vi "Auto Save Trigger Data.vi"(0 "Samples Recorded":u32 format="%#.0f", 1 "Data Log Indicies":i32[](array[numeric]), 2 "Log Path Ref":refnum<file>, 3 "Config":T1={"DAQ Settings"={"Trigger Type"=enum."Manual", "Trigger Samples"=0, "Pretrigger Samples"=0, "Trigger Interval"=0.0, "Time Units"=FALSE, "Auto Save"=FALSE, "Sample Rate"=7.0, "Select Analog"=FALSE, "Trigger Value"=0.0, "Trigger Stop Method"=enum."Use Samples Value to Stop Trigger", "Rate Sec/Min"=FALSE, "Save Mode"=enum."Single File", "File Size Limit"=0.0, "Log File Type"=enum."Basic", "Trigger Data Index"=0, "Log Rate"=7.0, "Rate Sec/Min (Log)"=FALSE, "Sample Rate (S/s)"=0.0, "Log Rate (S/s)"=0.0}, "Channels"=[], "Header"={"CA Number"="", "Test Name"="", "Serial Number"="", "Technician"=""}, "Graph Settings"={"Graph Labels"=[], [], [], [], [], [], [], [], [], [], [], [], [], "Graph Toggles"=[], "Axis Toggles"=[], "Graph Range"=enum."1"}, "Test Limits"=[], "All Type Info"=[], "Save Mode"=enum."Single File", "Data Base Path"=path ""} {"DAQ Settings"."Trigger Interval" min=0.0; "DAQ Settings"."Pretrigger Samples" min=0; "DAQ Settings"."Trigger Samples" min=0}, 4 "Data":sgl[][](array[numeric]), 5 "Start Time":timestamp, 6 "Add Data Point":bool, 7 "Samples Acquired":u32, 11 "Pretrigger Size":i32) -> (14 "Samples Recorded OUT":u32, 18 "Stop DAQ":bool, 19 "Samples Acquired OUT":u32)   [LabVIEW 2023]
uses:
  Type Defs and Controls/Sensor Config.ctl
  Type Defs and Controls/DAQ Settings.ctl
  Type Defs and Controls/Trigger Stop Method.ctl
  Type Defs and Controls/Log File Type.ctl
  Type Defs and Controls/Channel Config.ctl
  Type Defs and Controls/Header.ctl
  Type Defs and Controls/Graph Settings Type Def.ctl
  Type Defs and Controls/Test Limits.ctl
  Type Defs and Controls/All Part Info.ctl
  Type Defs and Controls/Part Info.ctl
panel:
  # "EGU"
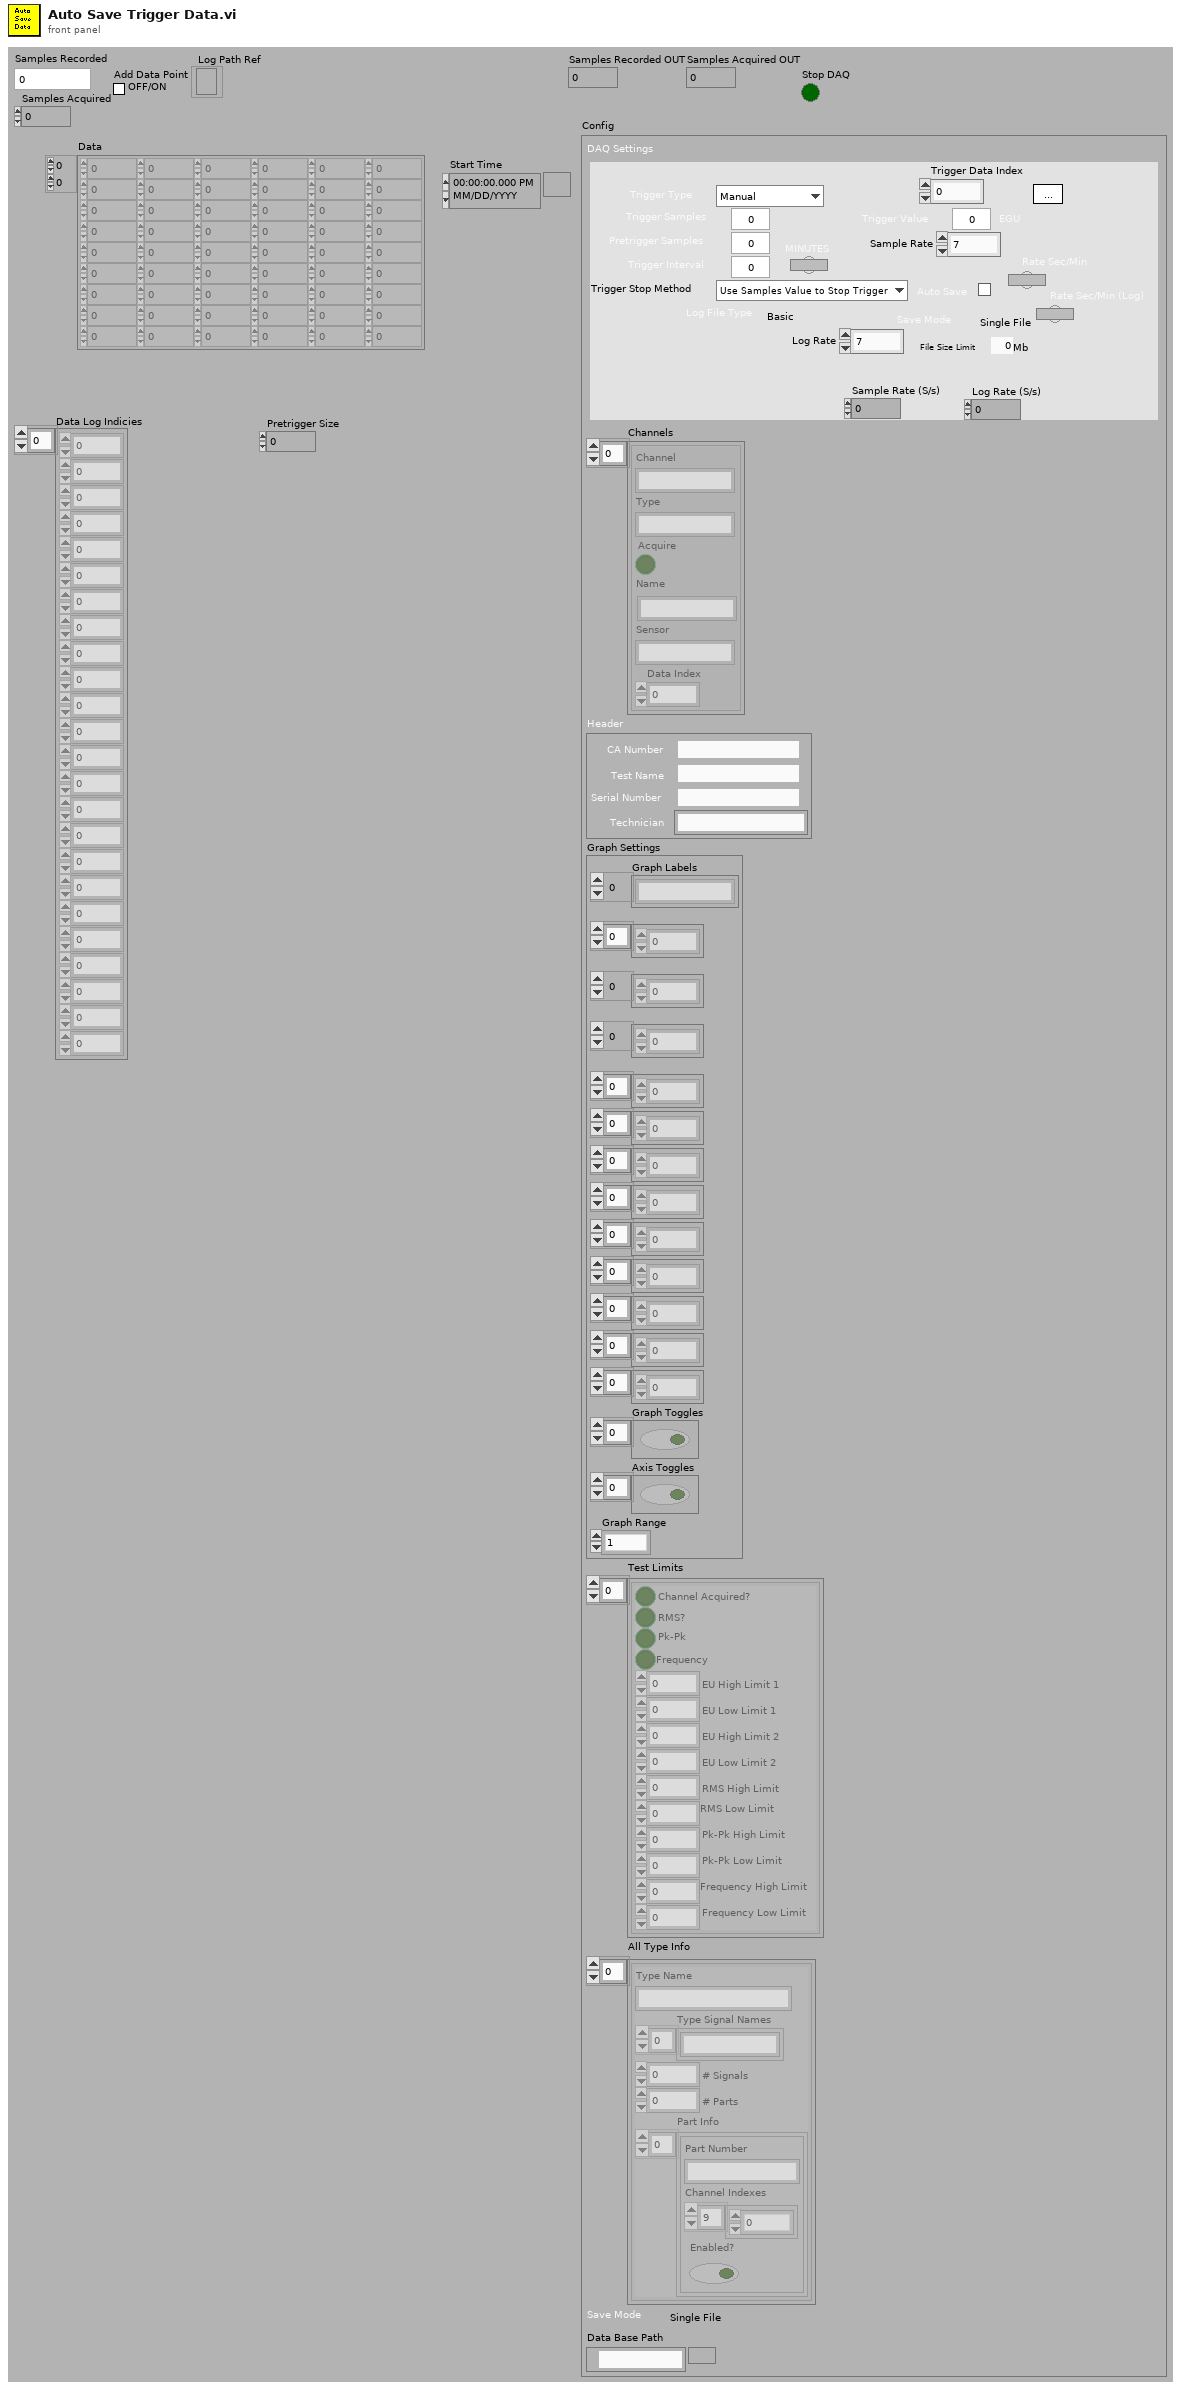
[diagram p1: front panel]
types:
  T1 = typedef "Sensor Config.ctl" = cluster{"DAQ Settings":T2, "Channels":T5[], "Header":T6, "Graph Settings":T7, "Test Limits":T8[], "All Type Info":T9, "Save Mode":enum16{"Single File", "Segmented Files", "New File at Midnight"}, "Data Base Path":path}
  T2 = typedef "DAQ Settings.ctl" = cluster{"Trigger Type":enum16{"Manual", "Timed", "Analog Rising", "Analog Falling"}, "Trigger Samples":i32, "Pretrigger Samples":i32, "Trigger Interval":dbl, "Time Units":bool, "Auto Save":bool, "Sample Rate":dbl, "Select Analog":bool, "Trigger Value":dbl, "Trigger Stop Method":T3, "Rate Sec/Min":bool, "Save Mode":enum16{"Single File", "Segmented Files", "New File at Midnight"}, "File Size Limit":dbl, "Log File Type":T4, "Trigger Data Index":u32, "Log Rate":dbl, "Rate Sec/Min (Log)":bool, "Sample Rate (S/s)":dbl, "Log Rate (S/s)":dbl}
  T3 = typedef "Trigger Stop Method.ctl" = enum16{"Use Samples Value to Stop Trigger", "Use Threshold to Stop Trigger"}
  T4 = typedef "Log File Type.ctl" = enum16{"Basic", "RTS"}
  T5 = typedef "Channel Config.ctl" = cluster{"Channel":string, "Type":string, "Acquire":bool, "Name":string, "Sensor":string, "Data Index":u32}
  T6 = typedef "Header.ctl" = cluster{"CA Number":string, "Test Name":string, "Serial Number":string, "Technician":string}
  T7 = typedef "Graph Settings Type Def.ctl" = cluster{"Graph Labels":string[], u8[], i16[], u32[], u8[], u8[], u8[], u32[], u8[], u8[], u8[], dbl[], dbl[], "Graph Toggles":bool[], "Axis Toggles":bool[], "Graph Range":enum16{"1", "2", "3", "4", "5", "10", "15", "30", "60"}}
  T8 = typedef "Test Limits.ctl" = cluster{"Channel Acquired?":bool, "RMS?":bool, "Pk-Pk":bool, "Frequency":bool, "EU High Limit 1":dbl, "EU Low Limit 1":dbl, "EU High Limit 2":dbl, "EU Low Limit 2":dbl, "RMS High Limit":dbl, "RMS Low Limit":dbl, "Pk-Pk High Limit ":dbl, "Pk-Pk Low Limit":dbl, "Frequency High Limit":dbl, "Frequency Low Limit":dbl}
  T9 = typedef "All Part Info.ctl" = cluster{"Type Name":string, "Type Signal Names":string[], "# Signals":i32, "# Parts":i32, "Part Info":T10[]}[]
  T10 = typedef "Part Info.ctl" = cluster{"Part Number":string, "Channel Indexes":u16[], "Enabled?":bool}
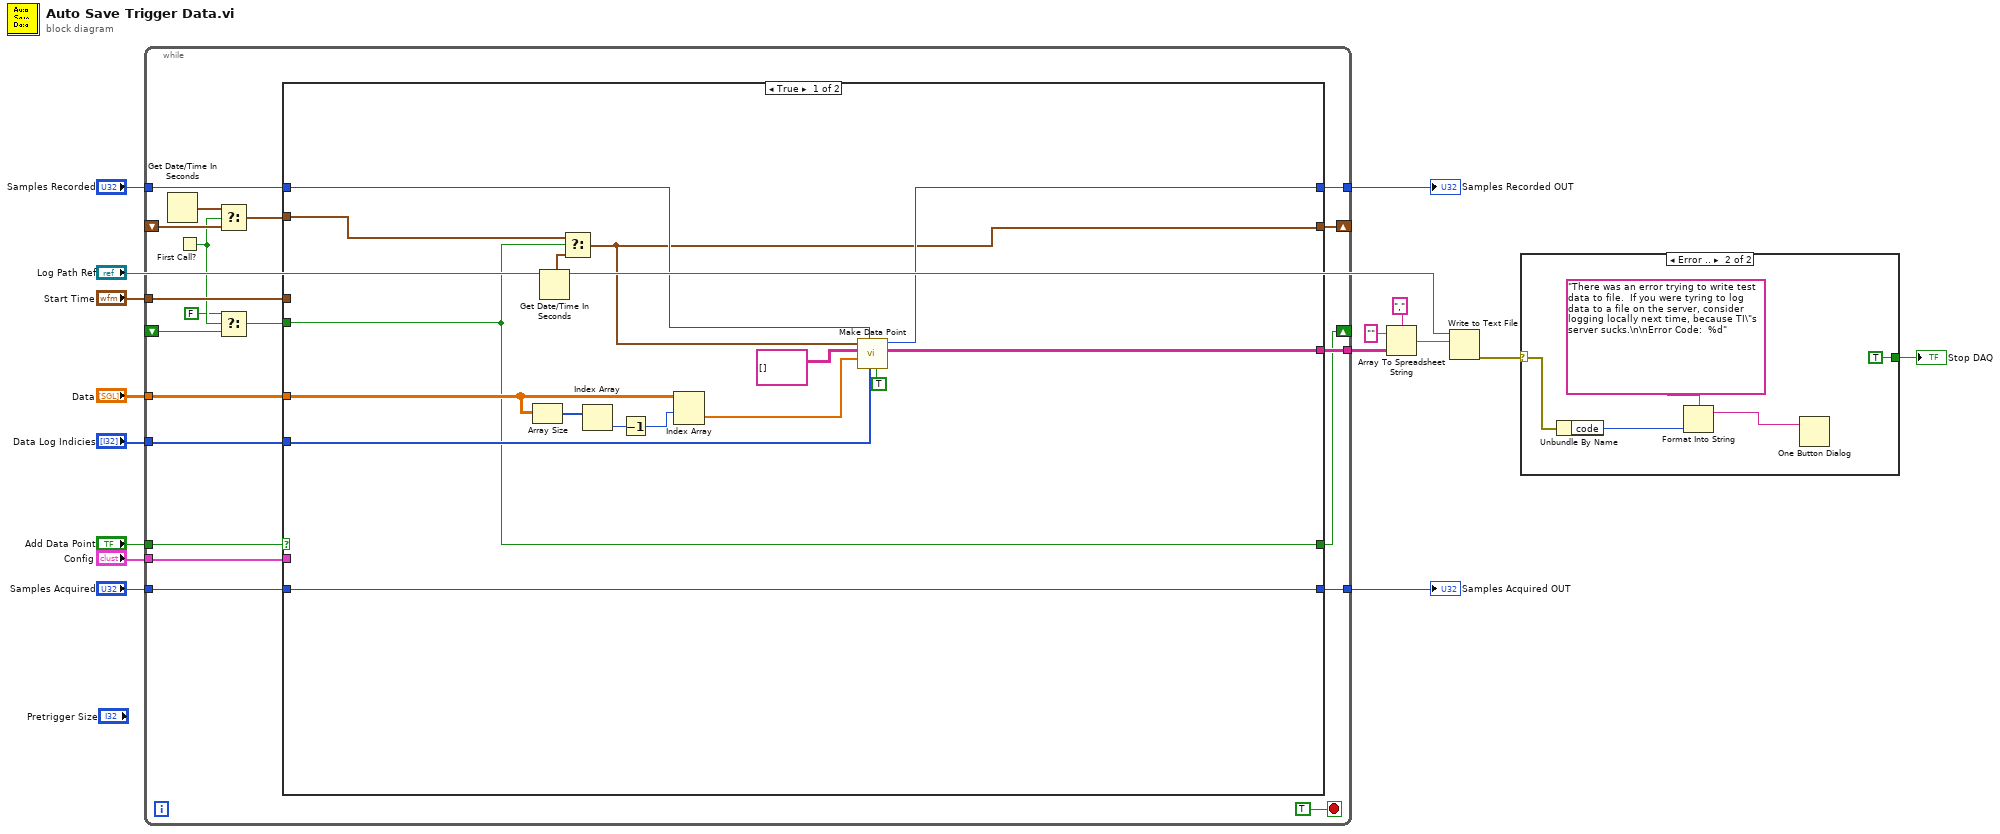
[diagram p0: block diagram]
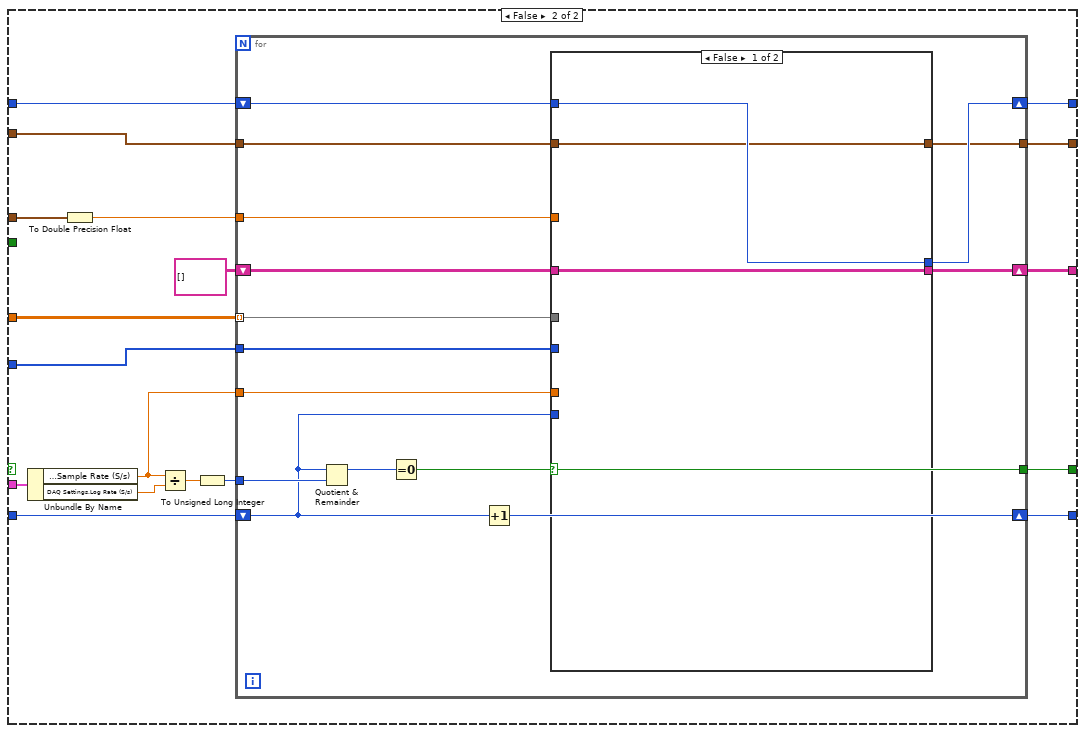
[diagram p2: hidden frame]
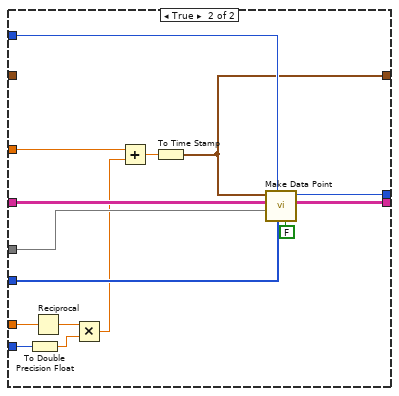
[diagram p3: hidden frame]
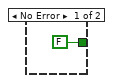
[diagram p4: hidden frame]
diagram:
  n1 = while {
    tunnel: "Config" -> [w36]
    tunnel: [w35] -> w6
    tunnel: "Data" -> [w34]
    tunnel: "Data Log Indicies" -> [w33]
    tunnel: "Samples Acquired" -> [w32]
    tunnel: "Samples Recorded" -> [w31]
    tunnel: [w30] -> w11
    tunnel: [w29] -> w10
    tunnel: "Start Time" -> [w28]
    shift-right: [w27] -> _
    shift-left: _ -> [w25]
    tunnel: "Add Data Point" -> [w22]
    shift-right: [w17] -> _
    shift-left: _ -> [w21]
    stop <- TRUE stop-if-true
    n2 = Get Date/Time In Seconds() -> (seconds since 1Jan1904=w23:timestamp)
    n3 = First Call?() -> (First Call?: T/F=w20:bool)
    n4 = Select(t=w23, s=w20, f=w25) -> (s? t:f=w24:timestamp)
    n5 = Select(t=FALSE ("First Call?: T/F"), s=w20, f=w21) -> (s? t:f=w18:bool)
    n6 = case shown="True" w22 {
      tunnel: w36 -> [_ w70]
      tunnel: [w52 w69] -> w35
      tunnel: w34 -> [w45 w67]
      tunnel: w33 -> [w51 w66]
      tunnel: w32 -> [w47 w63]
      tunnel: w31 -> [w48 w61]
      tunnel: [w50 w60] -> w30
      tunnel: [w47 w59] -> w29
      tunnel: w28 -> [_ w58]
      tunnel: [w39 w55] -> w27
      tunnel: [w38 w54] -> w17
      tunnel: w24 -> [w40 w53]
      tunnel: w18 -> [w38 _]
      frame True {
        n7 = Array Size(array=w45) -> (size(s)=w44:i32[])
        n8 = Get Date/Time In Seconds() -> (seconds since 1Jan1904=w37:timestamp)
        n9 = Select(t=w40, s=w38, f=w37) -> (s? t:f=w39:timestamp)
        n10 = Index Array(array=w44) -> (element=w42:i32)  [unwired: 1 in]
        n11 = Decrement(x=w42) -> (x-1=w41:i32)
        n12 = Index Array(array=w45, index (row)=w41) -> (element=w43:sgl[])  [unwired: 1 in]
        n13 = call "Make Data Point.vi"("Add Data Point (F)"=TRUE, "Data Log Indicies"=w51, "Samples Recorded"=w48, "Data"=w43, "Array in"=string[][] [], "Start Time"=w39) -> ("Array out"=w52:string[][], "Samples Recorded"=w50:u32)  [unwired: 4 in]
      }
      frame False {
        n14 = Unbundle By Name(w70) -> ("DAQ Settings.Sample Rate (S/s)"=w56:dbl, "DAQ Settings.Log Rate (S/s)"=w65:dbl)
        n15 = To Double Precision Float(number=w58) -> (double precision float=w57:dbl)
        n16 = Divide(x=w56, y=w65) -> (x/y=w64:dbl)
        n17 = To Unsigned Long Integer(number=w64) -> (unsigned 32bit integer=w62:u32)
        n18 = for {
          shift-right: [w75] -> w69
          shift-left: string[][] [] -> [w85]
          tunnel: w67 -> [w76] mode=indexing
          tunnel: w66 -> [w77]
          tunnel: w62 -> [w84]
          shift-right: [w83] -> w59
          shift-left: w63 -> [w79]
          shift-right: [w74] -> w60
          shift-left: w61 -> [w82]
          tunnel: w57 -> [w81]
          tunnel: w56 -> [w80]
          tunnel: [w73] -> w55
          tunnel: [w72] -> w54
          tunnel: w53 -> [w71]
          n19 = Quotient & Remainder(x=w79, y=w84) -> (x-y*floor(x/y)=w78:u32)  [unwired: 1 out]
          n20 = Equal To 0?(x=w78) -> (x = 0?=w72:bool)
          n21 = Increment(x=w79) -> (x+1=w83:u32)
          n22 = case shown="False" w72 {
            tunnel: [w88 w103] -> w75
            tunnel: w85 -> [w88 w102]
            tunnel: w76 -> [_ w101]
            tunnel: w77 -> [_ w100]
            tunnel: w82 -> [w87 w99]
            tunnel: w81 -> [_ w94]
            tunnel: w80 -> [_ w98]
            tunnel: w79 -> [_ w96]
            tunnel: [w87 w91] -> w74
            tunnel: [w86 w89] -> w73
            tunnel: w71 -> [w86 _]
            frame False {
            }
            frame True {
              n23 = To Double Precision Float(number=w96) -> (double precision float=w95:dbl)
              n24 = Reciprocal(x=w98) -> (1/x=w97:dbl)
              n25 = Multiply(x=w97, y=w95) -> (x*y=w93:dbl)
              n26 = Add(x=w94, y=w93) -> (x+y=w92:dbl)
              n27 = To Time Stamp(1:w92) -> (0:w89:timestamp)
              n28 = call "Make Data Point.vi"("Add Data Point (F)"=FALSE, "Data Log Indicies"=w100, "Samples Recorded"=w99, "Data"=w101, "Array in"=w102, "Start Time"=w89) -> ("Array out"=w103:string[][], "Samples Recorded"=w91:u32)  [unwired: 4 in]
            }
          }
        }
      }
    }
  }
  "Samples Recorded OUT" <- w11
  "Samples Acquired OUT" <- w10
  n29 = Array To Spreadsheet String(delimiter (Tab)=",", array=w6, 3:"" ("format string")) -> (spreadsheet string=w3:string)
  n30 = Write to Text File(file (use dialog)="Log Path Ref", text=w3) -> (error out=w1:errorcluster)  [unwired: 2 in, 2 out]
  n31 = case shown="Error .." w1 {
    selector: w1 -> [_ w108]
    tunnel: [FALSE TRUE] -> w8
    frame No Error {
    }
    frame Error {
      n32 = Unbundle By Name(w108) -> ("code"=w106:i32)
      n33 = Format Into String(format string="There was an error trying to write test data to file.  If you were tyring to log data to a file on the server, consider logging locally next time, because TI\"s server sucks.\n\nError Code:  %d" ("message"), w106) -> (resulting string=w105:string)  [unwired: 2 in, 1 out]
      n34 = One Button Dialog(message=w105) -> ()  [unwired: 1 in, 1 out]
    }
  }
  "Stop DAQ" <- w8
